vi "addapt error size.vi"(5 "stepsize":i32=10, 6 "Splitter":refnum<vi>, 7 "milliseconds to wait":u32, 9 "Pane in":refnum<vi>, 10 "String":refnum<vi>, 11 "VI in":refnum<vi>) -> ()   [LabVIEW 2013]
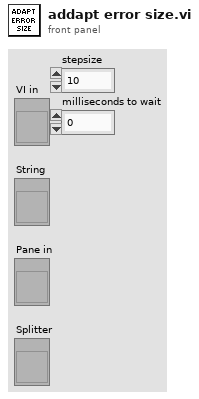
[diagram p1: front panel]
types:
  T1 = enum16{"Sticks Top/Left", "Sticks Bottom/Right", "Proportional"}
  T2 = typedef "LVRectTypeDef.ctl" = cluster{"Left":i16, "Top":i16, "Right":i16, "Bottom":i16}
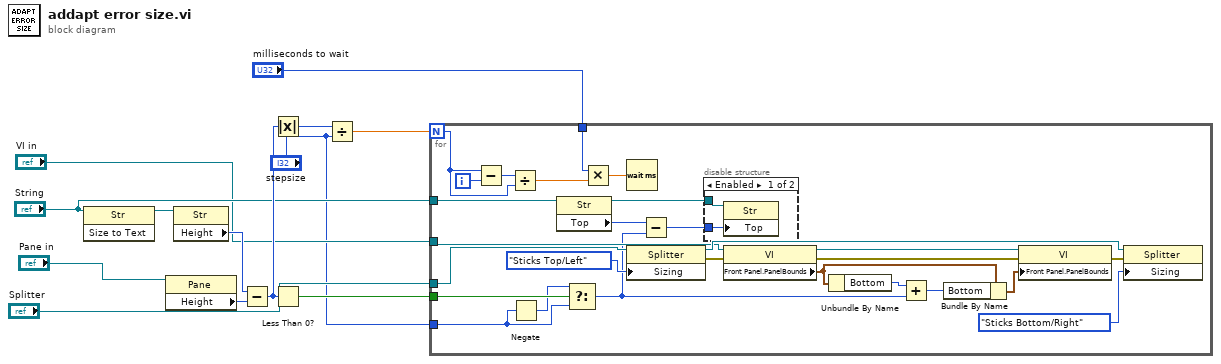
[diagram p0: block diagram]
diagram:
  n1 = invoke class="Str" method="Size to Text"(reference="String") -> (reference out=w7:refnum<vi>)  [unwired: 2 in, 2 out]
  n2 = property class="Pane"(reference="Pane in") -> ("Height"=w10:u32)  [unwired: 1 in, 2 out]
  n3 = property class="Str"(reference=w7) -> ("Height"=w9:u32)  [unwired: 1 in, 2 out]
  n4 = Subtract(x=w9, y=w10) -> (x-y=w13:i32)
  n5 = Absolute Value(x=w13) -> (abs(x)=w12:i32)
  n6 = Less Than 0?(x=w13) -> (x < 0?=w11:bool)
  n7 = Divide(x=w12, y="stepsize") -> (x/y=w5:dbl)
  n8 = for {
    N: w5 -> [w23]
    tunnel: "Splitter" -> [w35]
    tunnel: w11 -> [w28]
    tunnel: "VI in" -> [w26]
    tunnel: "String" -> [w20]
    tunnel: "stepsize" -> [w15]
    tunnel: "milliseconds to wait" -> [w14]
    i -> [w25]
    n9 = Subtract(x=w23, y=w25) -> (x-y=w24:i32)
    n10 = Divide(x=w24, y=w23) -> (x/y=w22:dbl)
    n11 = Negate(x=w15) -> (-x=w27:i32)
    n12 = property class="Str"(reference=w20) -> (reference out=w19:refnum<vi>, "Top"=w18:i32)  [unwired: 1 in, 1 out]
    n13 = Select(t=w27, s=w28, f=w15) -> (s? t:f=w17:i32)
    n14 = Multiply(x=w14, y=w22) -> (x*y=w21:dbl)
    n15 = Wait (ms)(milliseconds to wait=w21) -> ()  [unwired: 1 out]
    n16 = property class="Splitter"(reference=w35, "Sizing"=T1."Sticks Top/Left") -> (reference out=w30:refnum<vi>, error out=w34:errorcluster)  [unwired: 1 in]
    n17 = Subtract(x=w18, y=w17) -> (x-y=w16:i32)
    n18 = disable-structure shown="Enabled" {
      disable-tunnel: w19 -> [w42 _]
      disable-tunnel: w16 -> [w41 _]
      frame Enabled {
        n19 = property class="Str"(reference=w42, "Top"=w41) -> ()  [unwired: 1 in, 2 out]
      }
      frame Disabled {
      }
    }
    n20 = property class="VI"(reference=w26, error in=w34) -> (reference out=w40:refnum<vi>, error out=w32:errorcluster, "Front Panel.PanelBounds"=w39:T2)
    n21 = Unbundle By Name(w39) -> ("Bottom"=w38:i16)
    n22 = Add(x=w38, y=w17) -> (x+y=w37:i32)
    n23 = Bundle By Name(cluster=w39, "Bottom"=w37) -> (w36:T2)
    n24 = property class="VI"(reference=w40, error in=w32, "Front Panel.PanelBounds"=w36) -> (error out=w31:errorcluster)  [unwired: 1 out]
    n25 = property class="Splitter"(reference=w30, error in=w31, "Sizing"=T1."Sticks Bottom/Right") -> ()  [unwired: 2 out]
  }
